vi "simx Transfer File.vi"(6 "operationMode":i32, 7 "timeOut":i32, 8 "error in (no error)":errorcluster, 9 "fileName_serverSide":string, 10 "filePathAndName":string, 11 "clientID":i32) -> (0 "error out":errorcluster, 3 "function return":i32)   [LabVIEW 2019, in "PXL_V-REP.lvlib"]
doc: "EXTAPI_DLLEXPORT simxInt simxTransferFile(simxInt clientID,const simxChar* filePathAndName,const simxChar* fileName_serverSide,simxInt timeOut,simxInt operationMode);"
uses:
  PXL_V-REP.lvlib
  <userlib>/V-REP/remoteApi.dll
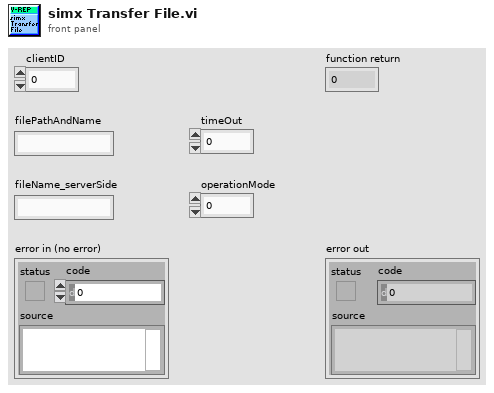
[diagram p1: front panel]
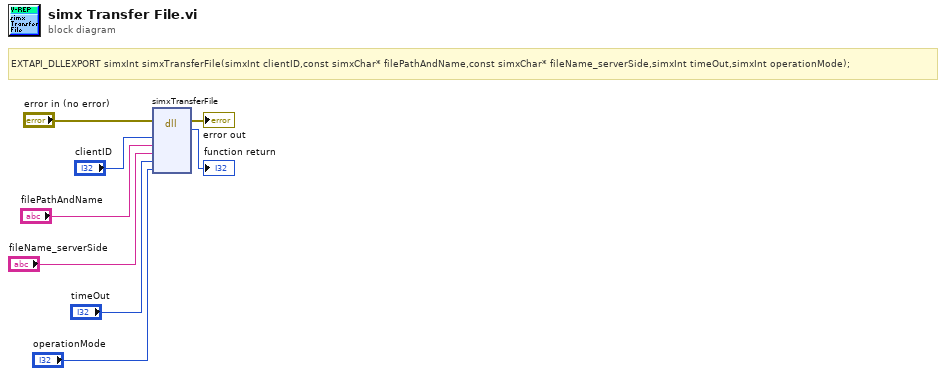
[diagram p0: block diagram]
diagram:
  # "EXTAPI_DLLEXPORT simxInt simxTransferFile(simxInt clientID,const simxChar* filePathAndName,const simxChar* fileName_serverSide,simxInt timeOut,simxInt operationMode);"
  n1 = dll-call lib="C:/Program Files (x86)/National Instruments/LabVIEW 2019/user.lib/V-REP/remoteApi.*" fn="simxTransferFile"(error in="error in (no error)", "clientID"="clientID", "filePathAndName"="filePathAndName", "fileName_serverSide"="fileName_serverSide", "timeOut"="timeOut", "operationMode"="operationMode") -> (error out=→"error out":errorcluster, →"function return":i32)  [unwired: 7 in, 1 out]
